vi "SimpleGetSpectrumExample.vi"() -> ()   [LabVIEW 2016]
doc: "This example VI demonstrates the use of the #GetSpectrum command to retrieve spectral data from Hyperion instruments.s"
uses:
  h.Library/COMM/CTL/h.COMM.Socket Type.ctl
  h.Library.lvlib
panel:
  out "Time Stamp (ns)":u64
  out "SN":u64
  out "Spectral Plots":cluster{dbl[], "Spectrum, db":dbl[]}[](graph)
  in  "Channel":u8=1 min=1 max=16 step=1
  in  "Address":string="172.20.117.55"
  # "Hyperion Simple #GetSpectrum Example"
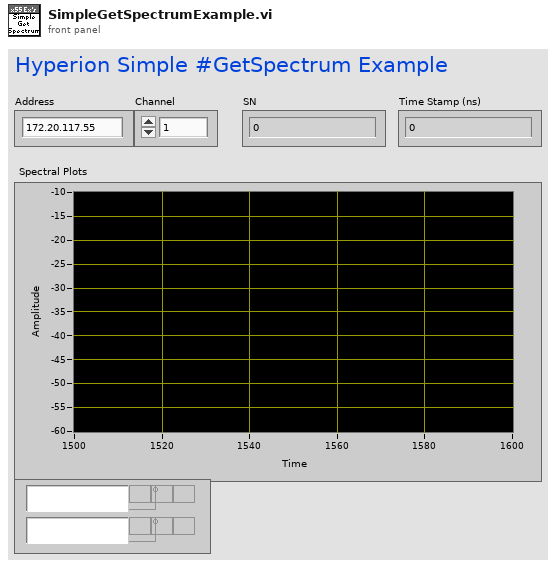
[diagram p1: front panel]
types:
  T1 = typedef "h.Library.lvlib/h.COMM.Socket Type.ctl" = u16
  T2 = typedef "h.Library.lvlib/h.ACQ.SpectralData.ctl" = cluster{"Spectrum":T3[], "Start Wvl":dbl, "Wvl Inc":dbl, "SN":u64, "Time Stamp (ns)":u64}
  T3 = typedef "h.Library.lvlib/h.ACQ.Spectrum.ctl" = cluster{"Spectrum, db":dbl[]}
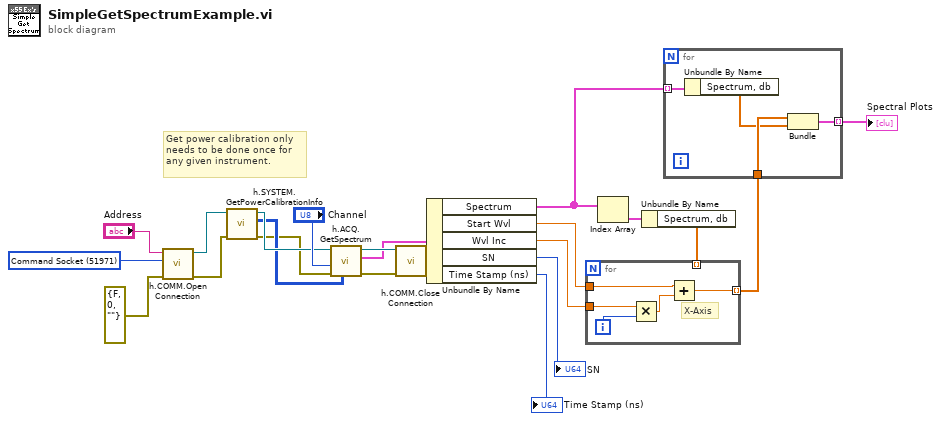
[diagram p0: block diagram]
diagram:
  w7 = T1 51971 items=["Command Socket"=51971, "Streaming Data Socket"=51972] ("Port")
  # "Get power calibration only\nneeds to be done once for\nany given instrument."
  n1 = call "h.COMM.Open Connection.vi"("error in"=errorcluster {"status"=FALSE, "code"=0, "source"=""}, "Port"=w7, "Address"="Address") -> ("error out"=w3:errorcluster, "Connection ID"=w6:refnum<k5>)  [unwired: 7 in]
  n2 = call "h.SYSTEM.GetPowerCalibrationInfo.vi"("error in"=w3, "Connection ID"=w6) -> ("error out"=w2:errorcluster, "power scales and offsets"=w4:i32[][], "Connection ID out"=w5:refnum<k5>)  [unwired: 7 in]
  n3 = call "h.ACQ.GetSpectrum.vi"("power scales and offsets"=w4, "error in"=w2, "Single Channel"="Channel", "Connection ID In"=w5) -> ("error out"=w1:errorcluster, "Spectral Data"=w17:T2, "Connection ID Out"=w19:refnum<k5>)  [unwired: 5 in]
  n4 = call "h.COMM.Close Connection.vi"("error in"=w1, "Connection ID"=w19) -> ()  [unwired: 9 in, 1 out]
  n5 = Unbundle By Name(w17) -> ("Spectrum"=w12:T3[], "Start Wvl"=w16:dbl, "Wvl Inc"=w15:dbl, "SN"=→"SN":u64, "Time Stamp (ns)"=→"Time Stamp (ns)":u64)
  n6 = Index Array(array=w12) -> (element=w14:T3)  [unwired: 1 in]
  n7 = Unbundle By Name(w14) -> ("Spectrum, db"=w13:dbl[])
  n8 = for {
    tunnel: w16 -> [w24]
    tunnel: w15 -> [w26]
    tunnel: [w22] -> w11 mode=indexing
    tunnel: w13 -> [_] mode=indexing
    i -> [w25]
    # "X-Axis"
    n9 = Multiply(x=w26, y=w25) -> (x*y=w23:dbl)
    n10 = Add(x=w24, y=w23) -> (x+y=w22:dbl)
  }
  n11 = for {
    tunnel: w12 -> [w30] mode=indexing
    tunnel: w11 -> [w29]
    tunnel: [w27] -> w10 mode=indexing
    n12 = Unbundle By Name(w30) -> ("Spectrum, db"=w28:dbl[])
    n13 = Bundle(w29, "Spectrum, db"=w28) -> (w27:cluster{dbl[], "Spectrum, db":dbl[]})  [unwired: 1 in]
  }
  "Spectral Plots" <- w10
